vi "Register Event.vi"   [LabVIEW 2019, in "GaitDAQ UI Event.lvlib"]
uses:
  GaitDAQ UI Event.lvlib
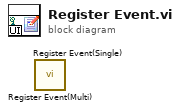
[diagram p0: block diagram]
diagram:
  n1 = call "Register Event(Multi).vi"() -> ()  [unwired: 11 in, 1 out]
  n2 = call "Register Event(Single).vi"() -> ()  [unwired: 11 in, 1 out]
